vi "name_of_caller.vi"(1 "is in inlined vi? (F)":bool, 3 "name of caller in":string) -> (0 "name of caller out":string)   [LabVIEW 2015]
doc: "Gives the name of the current vi's caller. If this vi is in inlied vi it gives the name of the calle one up the chain and so the 'is in inlined vi?' should be set to true. If, however, the name of caller up the chain is desired this is also a possible usage."
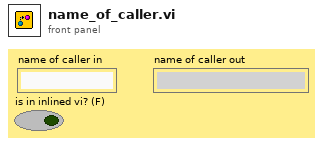
[diagram p1: front panel]
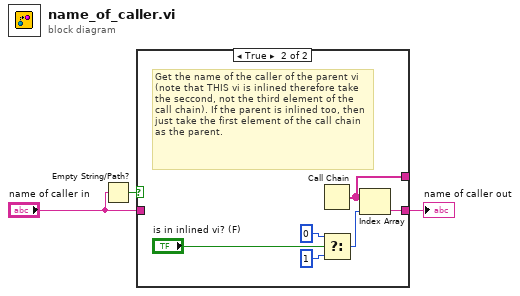
[diagram p0: block diagram]
diagram:
  n1 = Empty String/Path?(string/path="name of caller in") -> (empty?=w2:bool)
  n2 = case shown="True" w2 {
    tunnel: [w4 w10] -> w3
    tunnel: "name of caller in" -> [w4 _]
    tunnel: [_ w5] -> _
    frame False {
    }
    frame True {
      # "Get the name of the caller of the parent vi (note that THIS vi is inlined therefore take the seccond, not the third element of the call chain). If the parent is inlined too, then just take the first element of the call chain as the parent."
      n3 = Call Chain() -> (call chain=w5:string[])
      n4 = Select(t=0 ("index"), s="is in inlined vi? (F)", f=1 ("index")) -> (s? t:f=w6:i32)
      n5 = Index Array(array=w5, index=w6) -> (element=w10:string)
    }
  }
  "name of caller out" <- w3
